vi "OperatorID.vi"(3 "error in (no error)":errorcluster, 4 "OperatorLenth":i32=7, 5 "OperatorID":string) -> (0 "error out":errorcluster, 2 "OperatorIDOut":string)   [LabVIEW 2013]
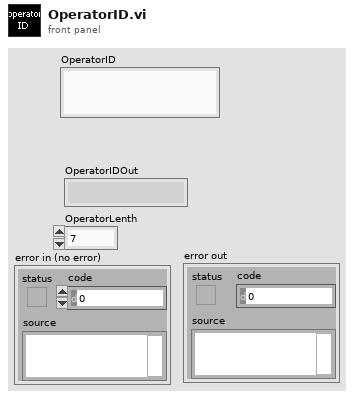
[diagram p1: front panel]
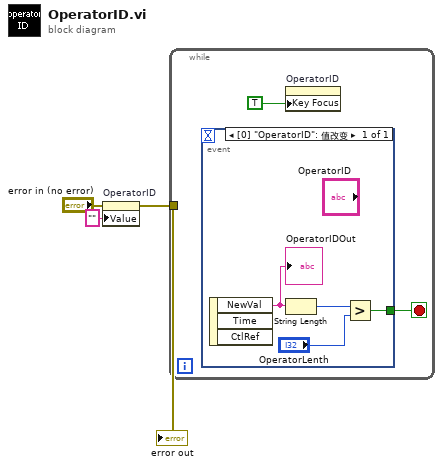
[diagram p0: block diagram]
diagram:
  n1 = property on="OperatorID" class="Str"(error in="error in (no error)", "Value"="" ("OperatorID")) -> (error out=w3:errorcluster)  [unwired: 1 in, 1 out]
  "error out" <- w3
  n2 = while {
    tunnel: w3 -> [_]
    stop <- w4 stop-if-true
    n3 = event shown="[0] \"OperatorID\": 值改变" {
      selector: _ -> [_]
      dyn-events: _ -> [_]
      timeout: _ -> [_]
      tunnel: [w6] -> w4
      event "OperatorID": Value Change {
        n4 = event-data() -> ("NewVal"=w8:string)  [unwired: 3 out]
        "OperatorIDOut" <- w8
        n5 = String Length(string=w8) -> (length=w9:i32)
        n6 = Greater?(x=w9, y="OperatorLenth") -> (0:w6:bool)
      }
    }
    n7 = property on="OperatorID" class="Str"("Key Focus"=TRUE) -> ()  [unwired: 2 in, 2 out]
  }
